vi "FTW-System-CPULoadAverage.vi"(5 "Minimum Measurement Period":dbl=0.1 format="%.3fsec", 7 "Maximum Measurement Period":dbl=10.0 format="%.3fsec", 11 "error in":errorcluster) -> (4 "Average Processor Utilization (Userspace)":dbl format="%.1f%%", 6 "Average Processor Utilization (System)":dbl format="%.1f%%", 8 "System Uptime":dbl format="%.3fmsec\n%<%D:%H:%M:%S%3u>t", 10 "Actual Measurement Period":dbl format="%.6fsec", 15 "error out":errorcluster)   [LabVIEW 2015]
panel:
  # "Inputs"
  # "Outputs"
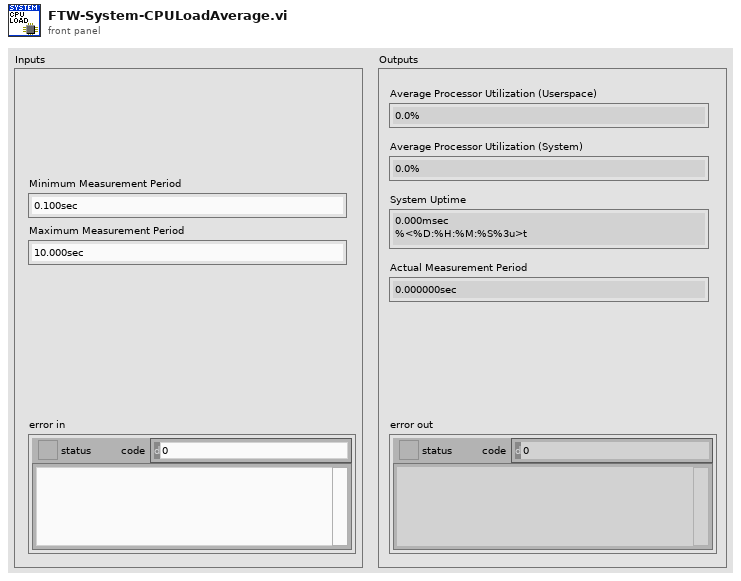
[diagram p1: front panel]
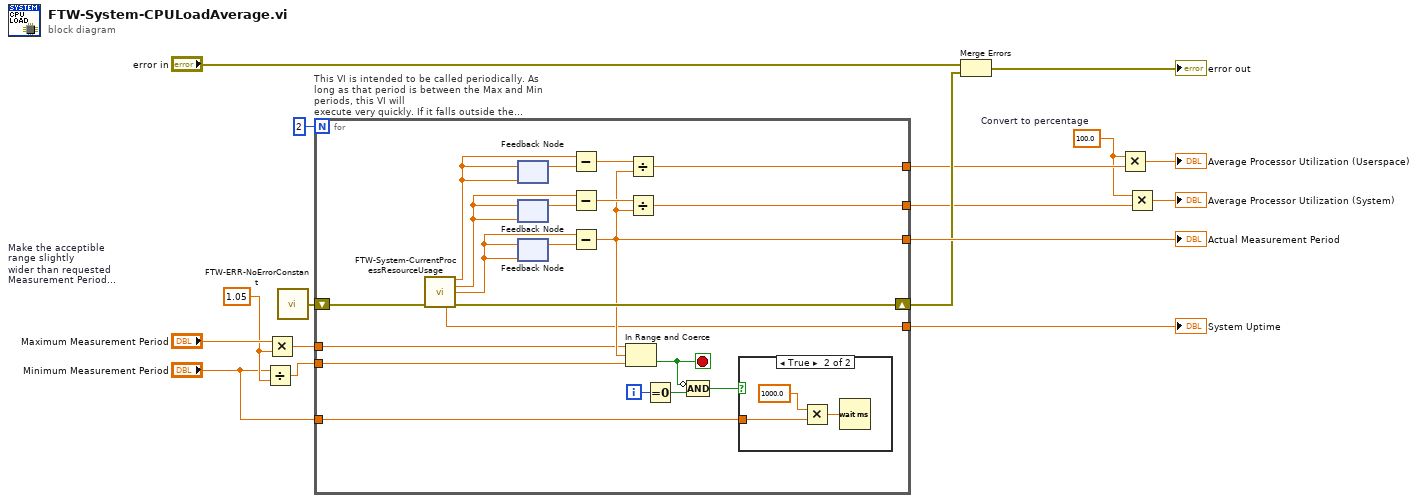
[diagram p0: block diagram]
diagram:
  w2 = 100.0  # Convert to percentage
  w9 = 1.05  # Make the acceptible range slightly wider than requested Measurement Period limits since sleeping is not a precise operation
  n1 = Divide(x="Minimum Measurement Period", y=w9) -> (x/y=w8:dbl)
  n2 = Multiply(x="Maximum Measurement Period", y=w9) -> (x*y=w10:dbl)
  n3 = call "FTW-ERR-NoErrorConstant.vi"() -> ("no error"=w14:errorcluster)
  n4 = for "This VI is intended to be called periodically. As long as that period is between the Max and Min periods, this VI will\nexecute very quickly. If it falls outside the range, this VI will block while waiting for the Minimum Measurement Period." {
    N: 2 -> [_]
    tunnel: [w30] -> w6
    tunnel: [w29] -> w3
    tunnel: [w26] -> w15
    shift-right: [w27] -> w12
    shift-left: w14 -> [w28]
    tunnel: w10 -> [w25]
    tunnel: w8 -> [w24]
    tunnel: "Minimum Measurement Period" -> [w19]
    tunnel: [w18] -> w1
    i -> [w23]
    stop <- w22 stop-if-true
    n5 = call "FTW-System-CurrentProcessResourceUsage.vi"("error in"=w28) -> ("Processor Time (Userspace)"=w33:dbl, "Processor Time (System)"=w32:dbl, "Current High-Resolution Timer"=w31:dbl, "System Uptime"=w18:dbl, "error out"=w27:errorcluster)  [unwired: 7 in, 3 out]
    n6 = feedback #1(w33) -> (w37:dbl)
    n7 = feedback-in #1(w33) -> ()
    n8 = feedback #2(w32) -> (w36:dbl)
    n9 = feedback-in #2(w32) -> ()
    n10 = feedback #3(w31) -> (w38:dbl)
    n11 = feedback-in #3(w31) -> ()
    n12 = Subtract(x=w33, y=w37) -> (x-y=w35:dbl)
    n13 = Subtract(x=w32, y=w36) -> (x-y=w34:dbl)
    n14 = Subtract(x=w31, y=w38) -> (x-y=w26:dbl)
    n15 = In Range and Coerce(upper limit=w25, x=w26, lower limit=w24) -> (In Range?=w22:bool)  [unwired: 1 out]
    n16 = Divide(x=w35, y=w26) -> (x/y=w30:dbl)
    n17 = Divide(x=w34, y=w26) -> (x/y=w29:dbl)
    n18 = Equal To 0?(x=w23) -> (x = 0?=w21:bool)
    n19 = Compound Arithmetic op=AND(invert w22, w21) -> (w20:bool)
    n20 = case shown="True" w20 {
      tunnel: w19 -> [_ w41]
      frame False {
      }
      frame True {
        n21 = Multiply(x=1000.0, y=w41) -> (x*y=w39:dbl)
        n22 = Wait (ms)(milliseconds to wait=w39) -> ()  [unwired: 1 out]
      }
    }
  }
  "Actual Measurement Period" <- w15
  "System Uptime" <- w1
  n23 = Merge Errors("error in", w12) -> (→"error out":errorcluster)
  n24 = Multiply(x=w2, y=w6) -> (x*y=→"Average Processor Utilization (Userspace)":dbl)
  n25 = Multiply(x=w2, y=w3) -> (x*y=→"Average Processor Utilization (System)":dbl)
